vi "Online Status.vi"(9 "MTX_DBO-B":bool, 10 "MTX-DBO-A":bool) -> (2 "UNIT ONLINE":string)   [LabVIEW 2019]
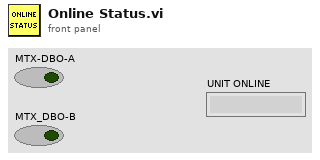
[diagram p1: front panel]
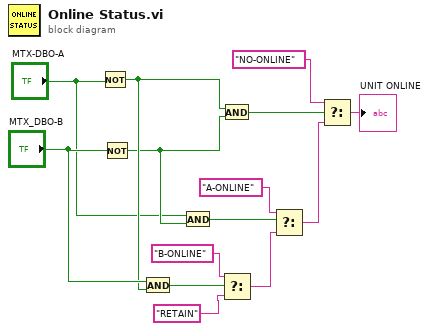
[diagram p0: block diagram]
diagram:
  n1 = Not(x="MTX-DBO-A") -> (.not. x?=w13:bool)
  n2 = Not(x="MTX_DBO-B") -> (.not. x?=w7:bool)
  n3 = And(x="MTX_DBO-B", y=w13) -> (x .and. y?=w8:bool)
  n4 = And(x="MTX-DBO-A", y=w7) -> (x .and. y?=w4:bool)
  n5 = And(x=w13, y=w7) -> (x .and. y?=w2:bool)
  n6 = Select(t="B-ONLINE", s=w8, f="RETAIN") -> (s? t:f=w10:string)
  n7 = Select(t="A-ONLINE", s=w4, f=w10) -> (s? t:f=w6:string)
  n8 = Select(t="NO-ONLINE", s=w2, f=w6) -> (s? t:f=→"UNIT ONLINE":string)
